vi "Set ForeColor.vi"(8 "error in":errorcluster, 10 "Color":refnum<class "Color.lvclass">, 11 "View in":refnum<class "Cell View.lvclass">) -> (0 "error out":errorcluster, 3 "View out":refnum<class "Cell View.lvclass">)   [LabVIEW 2024, in "SourceGrid.lvlib" / "Cell View.lvclass"]
uses:
  Cell View.lvclass
  Color/Color.lvclass
  Cell View.lvclass/Cell View.ctl
  Color/Color.lvclass/Color.ctl
  D:/git/Sourcegrid-LabVIEW/dll/SourceGrid.dll
  dll/SourceGrid.dll
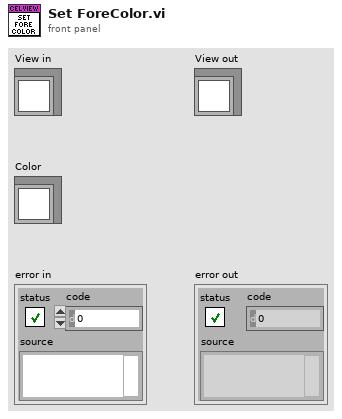
[diagram p1: front panel]
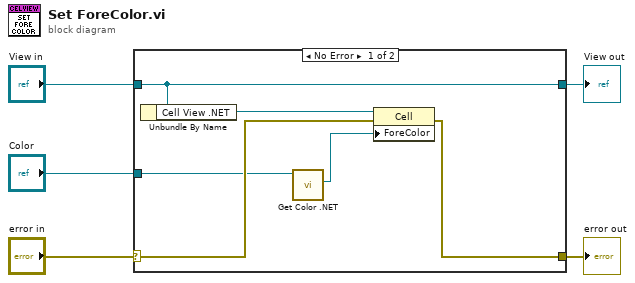
[diagram p0: block diagram]
diagram:
  n1 = case shown="No Error" "error in" {
    selector: "error in" -> [w10 w12]
    tunnel: [w7 w12] -> w4
    tunnel: [w6 w13] -> w2
    tunnel: "View in" -> [w6 w13]
    tunnel: "Color" -> [w9 _]
    frame No Error {
      n2 = Unbundle By Name(w6) -> ("Cell View .NET"=w11:refnum<k24>)
      n3 = call "Get Color .NET.vi"("Color in"=w9) -> ("Color .NET"=w8:refnum<k24>)  [unwired: 9 in, 1 out]
      n4 = property class="Cell"(reference=w11, error in=w10, "ForeColor"=w8) -> (error out=w7:errorcluster)  [unwired: 1 out]
    }
    frame Error {
    }
  }
  "error out" <- w4
  "View out" <- w2
